vi "Transmit Receive and Monitor All Channels.vi"() -> ()   [LabVIEW 2019]
doc: "This program opens the specified device, finds all cores with ARINC 429 channels, builds a transmit schedule using transmit interval information on all transmit channels, and configures all receive channels for monitoring. It also enables the Sequential Monitor to record transmitted and received messages."
uses:
  <instrlib>/BTI429Lib/Public/Controls/429 Record.ctl
  <instrlib>/BTICardLib/Private/Initialize By Card Number and Core Number.vi
  <instrlib>/BTICardLib/Private/Configure Core From XML.vi
  <instrlib>/BTI429Lib/Private/Tx/Configure/Configure Tx Channel From XML.vi
  <instrlib>/BTI429Lib/Private/Rx/Configure/Configure Rx Channel From XML.vi
  <instrlib>/BTI429Lib/Private/Core/Action-Status/Start All Channels.vi
  <instrlib>/BTI429Lib/Private/Core/Action-Status/Stop All Channels.vi
  <instrlib>/BTICardLib/BTICardLV.lvlib
  <instrlib>/BTI429Lib/BTI429LV.lvlib
panel:
  out "error out":errorcluster
  out "channelnumber":i32
  out "record out":T1 {"type" format="%04x"; "timestamp" format="%08x"; "msgact" format="%04x"; "data" format="%08x"; "timestamph" format="%08x"}
  in  "stop":bool
  in  "TX Channel XML Configuration XML file name":string="TX Channel Config.xml"
  in  "RX Channel XML Configuration XML file name":string="RX Channel Config.xml"
  in  "Core XML Configuration XML file name":string="Core Config.xml"
  in  "Card Number":i32
  # "ARINC 429: Transmit, Receive and Monitor All Channels"
  # "©2016 Astronics Ballard Technology"
  # "This program opens the specified device, finds all cores with ARINC 429 channels, builds a transmit schedule using transmit interval information on all transmit channels, and configures all receive channels for monitoring.  It also enables the Sequential Monitor to record transmitted and received messages."
  # "Always Stop the card\nand Close the card when\ndone. Otherwise, the hardware\ncontinues to operate."
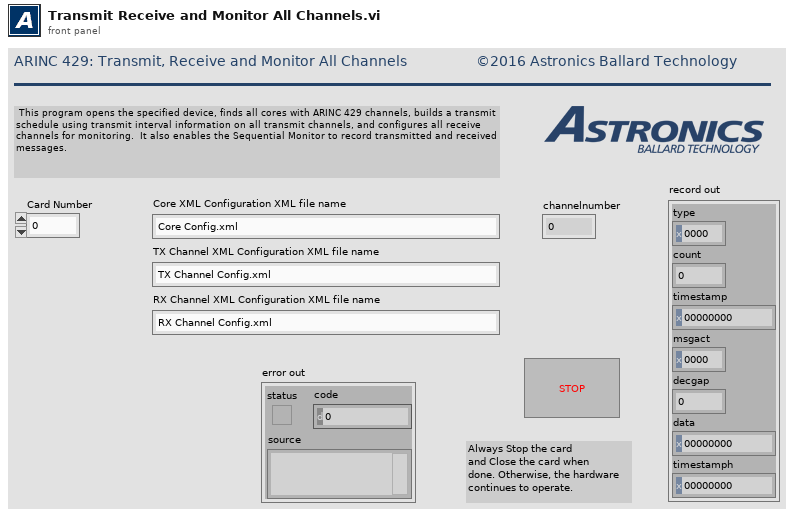
[diagram p1: front panel]
types:
  T1 = typedef "BTI429LV.lvlib/429 Record.ctl" = cluster{"type":u16, "count":u16, "timestamp":u32, "msgact":u16, "decgap":u16, "data":u32, "timestamph":u32}
  T2 = typedef "BTI429LV.lvlib/429 Activity Fields.ctl" = cluster{"channelnumber":i32, "speed":u32, "gaperror":bool, "parityerror":bool, "longworderror":bool, "bittimeerror":bool, "timeouterror":bool, "reserved":i8, "reserved":i8, "reserved":i8, "anyerror":bool, "hit":bool}
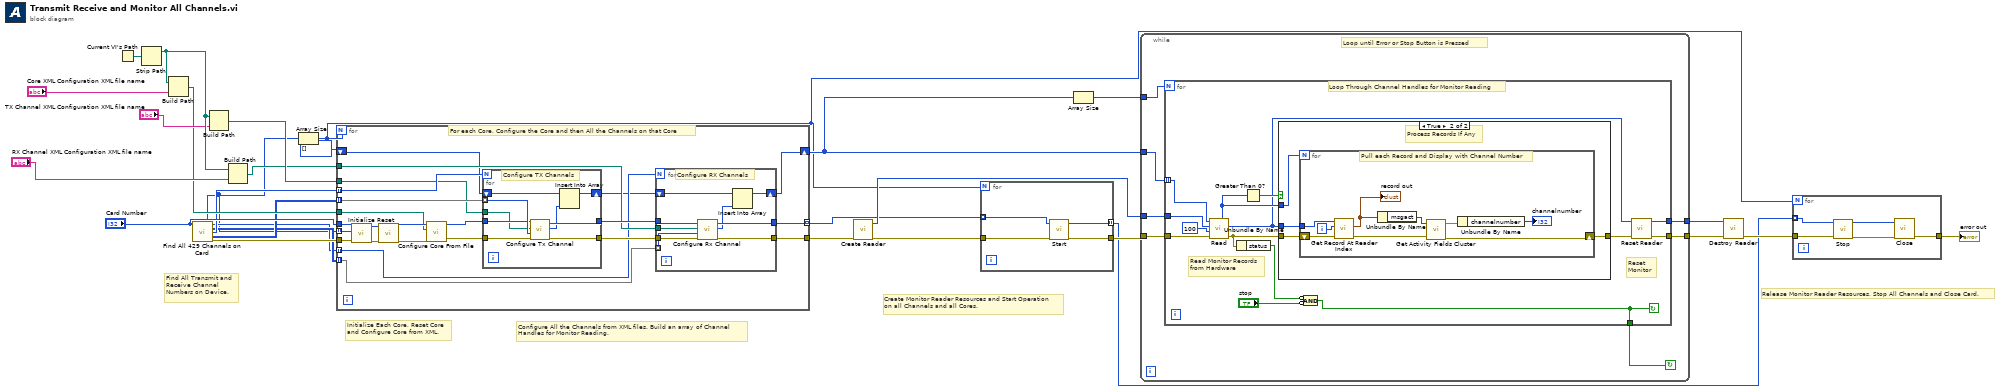
[diagram p0: block diagram]
diagram:
  # "Configure All the Channels from XML files. Build an array of Channel\nHandles for Monitor Reading."
  # "Create Monitor Reader Resources and Start Operation\non all Channels and all Cores."
  # "Release Monitor Reader Resources, Stop All Channels and Close Card."
  # "Initialize Each Core, Reset Core \nand Configure Core from XML."
  # "Find All Transmit and\nReceive Channel\nNumbers on Device."
  n1 = Current VI's Path() -> (path=w29:path)
  n2 = Strip Path(path=w29) -> (stripped path=w27:path)  [unwired: 1 out]
  n3 = Build Path(base path=w27, name or relative path="Core XML Configuration XML file name") -> (appended path=w24:path)
  n4 = call "Find All 429 Channels on Card.vi"("Card Number"="Card Number") -> ("Core Numbers"=w11:i32[], "Number of RX Channels"=w16:i32[], "Rx Channels"=w17:i32[][], "Number of TX Channels"=w20:i32[], "Tx Channels"=w21:i32[][], "error out"=w23:errorcluster)  [unwired: 9 in]
  n5 = Build Path(base path=w27, name or relative path="TX Channel XML Configuration XML file name") -> (appended path=w19:path)
  n6 = Build Path(base path=w27, name or relative path="RX Channel XML Configuration XML file name") -> (appended path=w18:path)
  n7 = Array Size(array=w11) -> (size(s)=w2:i32)
  n8 = for {
    N: w2 -> [_]
    tunnel: w24 -> [w48]
    tunnel: w23 -> [w47]
    tunnel: "Card Number" -> [w46]
    tunnel: w11 -> [w45] mode=indexing
    tunnel: w21 -> [w43] mode=indexing
    tunnel: w20 -> [w44] mode=indexing
    tunnel: w19 -> [w40]
    tunnel: w18 -> [w37]
    tunnel: w17 -> [w36] mode=indexing
    tunnel: w16 -> [w35] mode=indexing
    tunnel: [w34] -> w15
    tunnel: [w33] -> w7 mode=indexing
    shift-right: [w30] -> w8
    shift-left: u64[] [] -> [w32]
    # "For each Core, Configure the Core and then All the Channels on that Core"
    n9 = call-poly <instrlib>:"Initialize.vi"("error in (no error)"=w47, "core number"=w45, "card number"=w46) -> ("error out"=w51:errorcluster, "core handle out"=w52:u64)  [unwired: 7 in]
    n10 = call <instrlib>:"Reset.vi"("error in (no error)"=w51, "core handle in"=w52) -> ("error out"=w49:errorcluster, "core handle out"=w50:u64)  [unwired: 8 in]
    n11 = call-poly <instrlib>:"Configure Core From File.vi"("error in (no error)"=w49, "configuration file path"=w48, "core handle in"=w50) -> ("error out"=w41:errorcluster, "core handle out"=w42:u64)  [unwired: 7 in]
    n12 = for {
      N: w44 -> [_]
      tunnel: w43 -> [w70] mode=indexing
      tunnel: w42 -> [w69]
      tunnel: w41 -> [w68]
      tunnel: w40 -> [w67]
      tunnel: [w66] -> w39
      tunnel: [w65] -> w38
      shift-right: [w64] -> w31
      shift-left: w32 -> [w63]
      # "Configure TX Channels"
      n13 = call-poly <instrlib>:"Configure Tx Channel.vi"("error in (no error)"=w68, "channel number in"=w70, "configuration file path"=w67, "core handle in"=w69) -> ("error out"=w66:errorcluster, "channel handle out"=w62:u64, "core handle out"=w65:u64)  [unwired: 5 in]
      n14 = Insert Into Array(array=w63, new element=w62) -> (w64:u64[])  [unwired: 1 in]
    }
    n15 = for {
      N: w35 -> [_]
      tunnel: w39 -> [w61]
      tunnel: w38 -> [w60]
      tunnel: w37 -> [w59]
      tunnel: w36 -> [w58] mode=indexing
      tunnel: [w57] -> w34
      tunnel: [w56] -> w33
      shift-right: [w55] -> w30
      shift-left: w31 -> [w54]
      # "Configure RX Channels"
      n16 = call-poly <instrlib>:"Configure Rx Channel.vi"("error in (no error)"=w61, "channel number in"=w58, "configuration file path"=w59, "core handle in"=w60) -> ("error out"=w57:errorcluster, "channel handle out"=w53:u64, "core handle out"=w56:u64)  [unwired: 5 in]
      n17 = Insert Into Array(array=w54, new element=w53) -> (w55:u64[])  [unwired: 1 in]
    }
  }
  n18 = call <instrlib>:"Create Reader.vi"("error in (no error)"=w15) -> ("error out"=w14:errorcluster, "reader handle out"=w12:u64)  [unwired: 9 in]
  n19 = for {
    N: w2 -> [_]
    tunnel: w14 -> [w74]
    tunnel: [w73] -> w13
    tunnel: w7 -> [w72] mode=indexing
    tunnel: [w71] -> w1 mode=indexing
    n20 = call-poly <instrlib>:"Start.vi"("error in (no error)"=w74, "core handle in"=w72) -> ("error out"=w73:errorcluster, "core handle out"=w71:u64)  [unwired: 8 in]
  }
  n21 = Array Size(array=w8) -> (size(s)=w9:i32)
  n22 = while {
    tunnel: [w79] -> w5
    tunnel: w12 -> [w80]
    tunnel: w13 -> [w81]
    tunnel: [w78] -> w3
    tunnel: w8 -> [w77]
    tunnel: w9 -> [w76]
    stop <- w75 continue-if-true
    # "Loop until Error or Stop Button is Pressed"
    n23 = for {
      N: w76 -> [_]
      tunnel: w81 -> [w95]
      tunnel: w80 -> [w94]
      tunnel: [w93] -> w79
      tunnel: [w92] -> w78
      tunnel: w77 -> [w83] mode=indexing
      tunnel: [w82] -> w75
      stop <- w82 continue-if-true
      # "Reset\nMonitor"
      # "Read Monitor Records\nfrom Hardware"
      # "Loop Through Channel Handles for Monitor Reading"
      n24 = call <instrlib>:"Read.vi"("error in (no error)"=w95, "max records to read"=100, "reader handle in"=w94, "channel handle in"=w83) -> ("error out"=w85:errorcluster, "reader handle out"=w86:u64, "records read"=w87:i32)  [unwired: 3 in, 2 out]
      n25 = Unbundle By Name(w85) -> ("status"=w91:bool)
      n26 = Greater Than 0?(x=w87) -> (x > 0?=w88:bool)
      n27 = case shown="True" w88 {
        tunnel: w86 -> [_ w100]
        tunnel: w87 -> [_ w99]
        tunnel: w85 -> [w96 w97]
        tunnel: [w96 w98] -> w84
        frame False {
        }
        frame True {
          # "Process Records If Any"
          n28 = for {
            N: w99 -> [_]
            tunnel: w100 -> [w109]
            shift-right: [w103] -> w98
            shift-left: w97 -> [w107]
            i -> [w108]
            # "Pull each Record and Display with Channel Number"
            n29 = call <instrlib>:"Get Record At Reader Index.vi"("error in (no error)"=w107, "record index"=w108, "reader handle in"=w109) -> ("error out"=w104:errorcluster, "record out"=w106:T1)  [unwired: 6 in, 1 out]
            "record out" <- w106
            n30 = Unbundle By Name(w106) -> ("msgact"=w102:u16)
            n31 = call <instrlib>:"Get Activity Fields Cluster.vi"("error in (no error)"=w104, "msgact"=w102) -> ("error out"=w103:errorcluster, "fields cluster"=w105:T2)  [unwired: 8 in]
            n32 = Unbundle By Name(w105) -> ("channelnumber"=→"channelnumber":i32)
          }
        }
      }
      n33 = Compound Arithmetic op=AND(invert w91, invert "stop") -> (w82:bool)
      n34 = call <instrlib>:"Reset Reader.vi"("error in (no error)"=w84, "reader handle in"=w86) -> ("error out"=w93:errorcluster, "reader handle out"=w92:u64)  [unwired: 8 in]
    }
  }
  n35 = call <instrlib>:"Destroy Reader.vi"("error in (no error)"=w5, "reader handle in"=w3) -> ("error out"=w4:errorcluster)  [unwired: 8 in, 1 out]
  n36 = for {
    N: w2 -> [_]
    tunnel: [w113] -> w6
    tunnel: w4 -> [w111]
    tunnel: w1 -> [w110] mode=indexing
    n37 = call-poly <instrlib>:"Stop.vi"("error in (no error)"=w111, "core handle in"=w110) -> ("error out"=w114:errorcluster, "core handle out"=w112:u64)  [unwired: 8 in]
    n38 = call <instrlib>:"Close.vi"("error in (no error)"=w114, "core handle in"=w112) -> ("error out"=w113:errorcluster)  [unwired: 8 in, 1 out]
  }
  "error out" <- w6
